vi "Activate Port.vi"(8 "error in (no error)":errorcluster, 10 "data":T2, 11 "Message Handling Cluster":T1) -> (0 "error out":errorcluster, 3 "Message Handling Cluster":T1)   [LabVIEW 2024]
uses:
  Controls/Tab Enums/Activation Type Enum.ctl
  Controls/Clusters/Activate Port Cluster.ctl
  Controls/Clusters/Message Handling Cluster.ctl
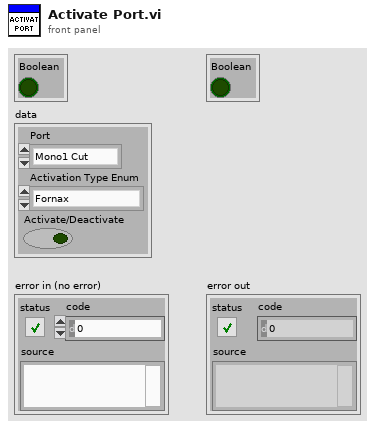
[diagram p1: front panel]
types:
  T1 = typedef "Message Handling Cluster.ctl" = cluster{"Boolean":bool}
  T2 = typedef "Activate Port Cluster.ctl" = cluster{"Port":enum16{"Mono1 Cut", "Mono1 Coag", "Mono2 Cut", "Mono2 Coag", "Mono2 Triverse", "Bipolar", "Ligasure"}, "Activation Type Enum":T3, "Activate/Deactivate":bool}
  T3 = typedef "Activation Type Enum.ctl" = enum16{"Fornax", "Handswitch", "Footswitch", "Triverse", "Auto Bipolar"}
  T4 = enum16{"Mono1 Cut", "Mono1 Coag", "Mono2 Cut", "Mono2 Coag", "Mono2 Triverse", "Bipolar", "Ligasure"}
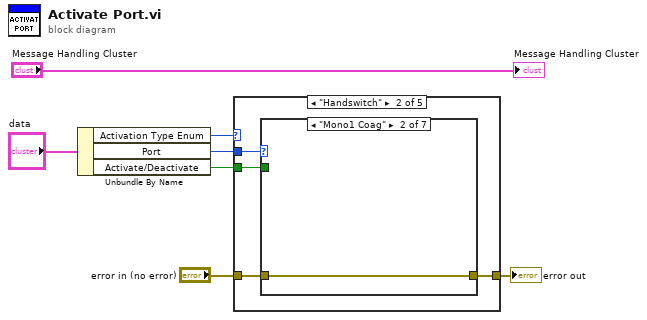
[diagram p0: block diagram]
diagram:
  n1 = Unbundle By Name("data") -> ("Activation Type Enum"=w2:T3, "Port"=w5:T4, "Activate/Deactivate"=w6:bool)
  n2 = case shown="\"Handswitch\"" w2 {
    tunnel: [w10 w21 w32 w43 w51] -> w4
    tunnel: "error in (no error)" -> [w9 w20 w31 w42 w50]
    tunnel: w5 -> [w11 w22 w33 w44 w52]
    tunnel: w6 -> [w8 w19 w30 w41 w49]
    frame "Fornax", Default {
      n3 = case shown="\"Mono1 Coag\"" w11 {
        tunnel: [w12 w13 w14 w15 w16 w17 w18] -> w10
        tunnel: w9 -> [w12 w13 w14 w15 w16 w17 w18]
        tunnel: w8 -> [_ _ _ _ _ _ _]
        frame "Mono1 Cut", Default {
        }
        frame "Mono1 Coag" {
        }
        frame "Mono2 Cut" {
        }
        frame "Mono2 Coag" {
        }
        frame "Mono2 Triverse" {
        }
        frame "Bipolar" {
        }
        frame "Ligasure" {
        }
      }
    }
    frame "Handswitch" {
      n4 = case shown="\"Mono1 Coag\"" w22 {
        tunnel: [w23 w24 w25 w26 w27 w28 w29] -> w21
        tunnel: w20 -> [w23 w24 w25 w26 w27 w28 w29]
        tunnel: w19 -> [_ _ _ _ _ _ _]
        frame "Mono1 Cut", Default {
        }
        frame "Mono1 Coag" {
        }
        frame "Mono2 Cut" {
        }
        frame "Mono2 Coag" {
        }
        frame "Mono2 Triverse" {
        }
        frame "Bipolar" {
        }
        frame "Ligasure" {
        }
      }
    }
    frame "Footswitch" {
      n5 = case shown="\"Mono1 Cut\", Default" w33 {
        tunnel: [w34 w35 w36 w37 w38 w39 w40] -> w32
        tunnel: w31 -> [w34 w35 w36 w37 w38 w39 w40]
        tunnel: w30 -> [_ _ _ _ _ _ _]
        frame "Mono1 Cut", Default {
        }
        frame "Mono1 Coag" {
        }
        frame "Mono2 Cut" {
        }
        frame "Mono2 Coag" {
        }
        frame "Mono2 Triverse" {
        }
        frame "Bipolar" {
        }
        frame "Ligasure" {
        }
      }
    }
    frame "Triverse" {
      n6 = case shown="Default" w44 {
        tunnel: [w45 w46 w47 w48] -> w43
        tunnel: w42 -> [w45 w46 w47 w48]
        tunnel: w41 -> [_ _ _ _]
        frame "Mono2 Cut" {
        }
        frame "Mono2 Coag" {
        }
        frame "Mono2 Triverse" {
        }
        frame Default {
        }
      }
    }
    frame "Auto Bipolar" {
      n7 = case shown="Default" w52 {
        tunnel: [w53 w54] -> w51
        tunnel: w50 -> [w53 w54]
        tunnel: w49 -> [_ _]
        frame "Bipolar" {
        }
        frame Default {
        }
      }
    }
  }
  "error out" <- w4
  "Message Handling Cluster" <- "Message Handling Cluster"
